vi "workbook set custom property number.vi"(8 "error in (no error)":errorcluster, 9 "value":dbl, 10 "name":string, 11 "workbook":u32) -> (0 "error out":errorcluster, 3 "function return":u32(ring))   [LabVIEW 2015, in "xlsxwriter.lvlib"]
doc: "lxw_error workbook_set_custom_property_number(lxw_workbook workbook, const char *name, double value);"
uses:
  xlsxwriter.lvlib
  xlsxwriter.dll
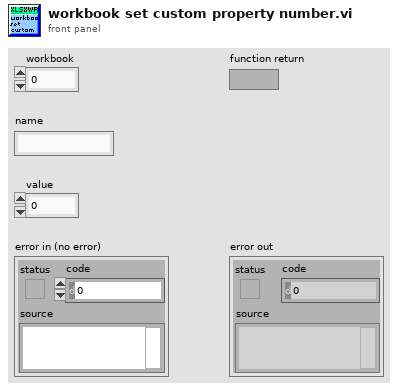
[diagram p1: front panel]
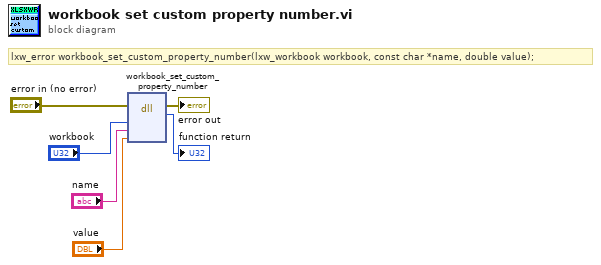
[diagram p0: block diagram]
diagram:
  # "lxw_error workbook_set_custom_property_number(lxw_workbook workbook, const char *name, double value);"
  n1 = dll-call lib="C:/Users/WDAGUtilityAccount/Desktop/lv_vis_added_cell/xlsxwriter.*" fn="workbook_set_custom_property_number"(error in="error in (no error)", "workbook"="workbook", "name"="name", "value"="value") -> (error out=→"error out":errorcluster, →"function return":u32)  [unwired: 5 in, 1 out]
